vi "analysis_speech01.vi"(11 "文件路径（使用对话框）":path) -> (2 "数组":dbl[](array[numeric]), 3 "波形图表":waveform(dbl)[](graph))   [LabVIEW 2014]
uses:
  <vilib>/sound2/lvsound2.llb/Sound File Read Open.vi
  <vilib>/sound2/lvsound2.llb/Sound File Read (DBL).vi
panel:
  in  "布尔":bool
  out "错误输出":errorcluster
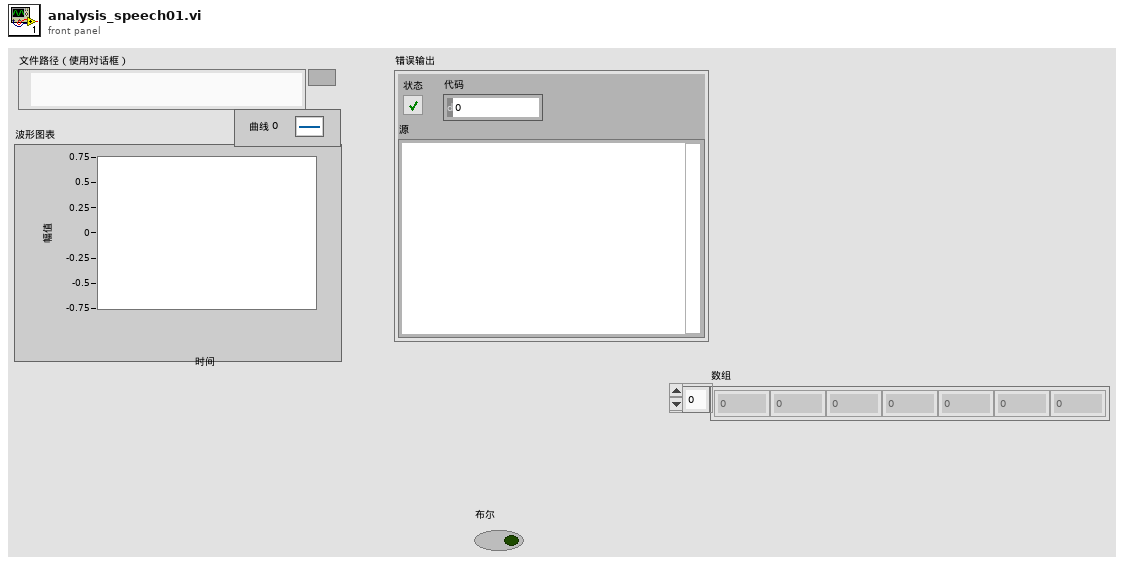
[diagram p1: front panel]
types:
  T1 = typedef "Sound File Refnum.ctl" = refnum<file>
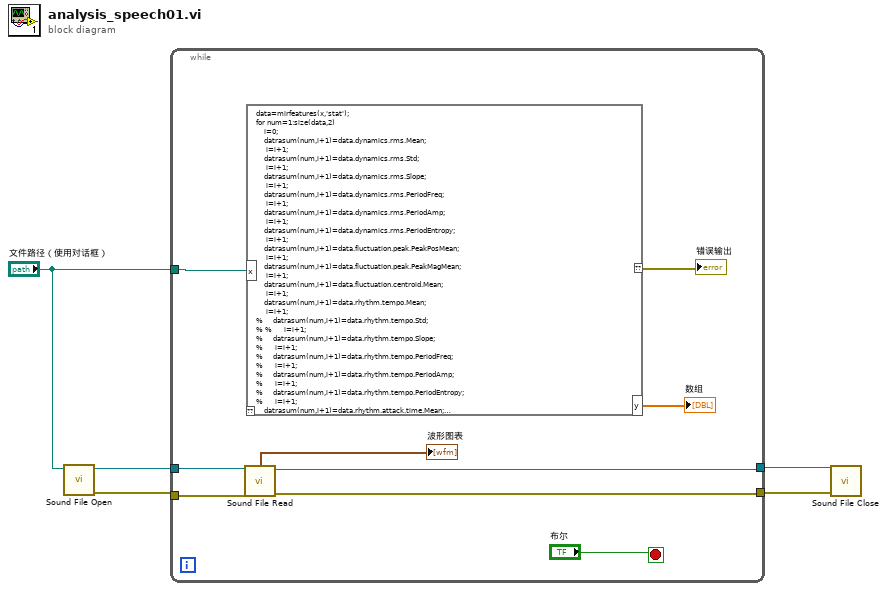
[diagram p0: block diagram]
diagram:
  n1 = call-poly <vilib>:"Sound File Open.vi"("path"="文件路径（使用对话框）") -> ("error out"=w2:errorcluster, "sound file refnum"=w4:T1)  [unwired: 9 in]
  n2 = while {
    tunnel: "文件路径（使用对话框）" -> [w10]
    tunnel: w4 -> [w11]
    tunnel: [w9] -> w3
    tunnel: w2 -> [w8]
    tunnel: [w7] -> w1
    stop <- "布尔" stop-if-true
    n3 = call-poly <vilib>:"Sound File Read.vi"("error in (no error)"=w8, "sound file refnum"=w11) -> ("error out"=w7:errorcluster, "data"=→"波形图表":waveform(dbl)[], "sound file refnum out"=w9:T1)  [unwired: 5 in, 2 out]
    n4 = script code="data=mirfeatures(x,'stat'); \nfor num=1:size(data,2)\n    i=0;\n    datrasum(num,i+1)=data.dynamics.rms.Mean;\n     i=i+1;\n    datrasum(num,i+1)=data.dynamics.rms.Std;\n     i=i+1;\n    datrasum(num,i+1)=data.dynamics.rms.Slope;\n     i=i+1;\n    datrasum(num,i+1)=data.dynamics.rms.PeriodFreq;\n     i=i+1;\n    datrasum(num,i+1)=data.dynamics.rms.PeriodAmp;\n     i=i+1;\n    datrasum(num,i+1)=data.dynamics.rms.PeriodEntropy;\n     i=i+1;\n    datrasum(num,i+1)=data.fluctuation.peak.PeakPosMean;\n     i=i+1;\n    datrasum(num,i+1)=data.fluctuation.peak.PeakMagMean;\n     i=i+1;\n    datrasum(num,i+1)=data.fluctuation.centroid.Mean;\n     i=i+1;\n    datrasum(num,i+1)=data.rhythm.tempo.Mean;\n     i=i+1;\n%     datrasum(num,i+1)=data.rhythm.tempo.Std;\n% %      i=i+1;\n%     datrasum(num,i+1)=data.rhythm.tempo.Slope;\n%      i=i+1;\n%     datrasum(num,i+1)=data.rhythm.tempo.PeriodFreq;\n%      i=i+1;\n%     datrasum(num,i+1)=data.rhythm.tempo.PeriodAmp;\n%      i=i+1;\n%     datrasum(num,i+1)=data.rhythm.tempo.PeriodEntropy;\n%      i=i+1;\n    datrasum(num,i+1)=data.rhythm.attack.time.Mean;\n     i=i+1;\n    datrasum(num,i+1)=data.rhythm.attack.time.Std;\n     i=i+1;\n    datrasum(num,i+1)=data.rhythm.attack.time.Slope;\n     i=i+1;\n    datrasum(num,i+1)=data.rhythm.attack.time.PeriodFreq;\n     i=i+1;\n    datrasum(num,i+1)=data.rhythm.attack.time.PeriodAmp;\n     i=i+1;\n    datrasum(num,i+1)=data.rhythm.attack.time.PeriodEntropy;\n     i=i+1;\n    datrasum(num,i+1)=data.rhythm.attack.slope.Mean;\n     i=i+1;\n    datrasum(num,i+1)=data.rhythm.attack.slope.Std;\n     i=i+1;\n    datrasum(num,i+1)=data.rhythm.attack.slope.Slope;\n     i=i+1;\n    datrasum(num,i+1)=data.rhythm.attack.slope.PeriodFreq;\n     i=i+1;\n    datrasum(num,i+1)=data.rhythm.attack.slope.PeriodAmp;\n     i=i+1;\n    datrasum(num,i+1)=data.rhythm.attack.slope.PeriodAmp;\n     i=i+1;\n    datrasum(num,i+1)=data.rhythm.attack.slope.PeriodEntropy;\n     i=i+1;\n    datrasum(num,i+1)=data.spectral.centroid.Mean;\n     i=i+1;\n    datrasum(num,i+1)=data.spectral.centroid.Std;\n     i=i+1;\n    datrasum(num,i+1)=data.spectral.centroid.Slope;\n     i=i+1;\n    datrasum(num,i+1)=data.spectral.centroid.PeriodFreq;\n     i=i+1;\n    datrasum(num,i+1)=data.spectral.centroid.PeriodAmp;\n     i=i+1;\n    datrasum(num,i+1)=data.spectral.centroid.PeriodEntropy;\n     i=i+1;\n    datrasum(num,i+1)=data.spectral.brightness.Mean;\n     i=i+1;\n    datrasum(num,i+1)=data.spectral.brightness.Std;\n     i=i+1;\n    datrasum(num,i+1)=data.spectral.brightness.Slope;\n     i=i+1;\n    datrasum(num,i+1)=data.spectral.brightness.PeriodFreq;\n     i=i+1;\n    datrasum(num,i+1)=data.spectral.brightness.PeriodAmp;\n     i=i+1;\n    datrasum(num,i+1)=data.spectral.brightness.PeriodEntropy;\n     i=i+1;\n    datrasum(num,i+1)=data.spectral.spread.Mean;\n     i=i+1;\n    datrasum(num,i+1)=data.spectral.spread.Std;\n     i=i+1;\n    datrasum(num,i+1)=data.spectral.spread.Slope;\n     i=i+1;\n    datrasum(num,i+1)=data.spectral.spread.PeriodFreq;\n     i=i+1;\n    datrasum(num,i+1)=data.spectral.spread.PeriodAmp;\n     i=i+1;\n    datrasum(num,i+1)=data.spectral.spread.PeriodEntropy;\n     i=i+1;\n    datrasum(num,i+1)=data.spectral.skewness.Mean;\n     i=i+1;\n    datrasum(num,i+1)=data.spectral.skewness.Std;\n     i=i+1;\n    datrasum(num,i+1)=data.spectral.skewness.Slope;\n     i=i+1;\n    datrasum(num,i+1)=data.spectral.skewness.PeriodFreq;\n     i=i+1;\n    datrasum(num,i+1)=data.spectral.skewness.PeriodAmp;\n     i=i+1;\n    datrasum(num,i+1)=data.spectral.skewness.PeriodEntropy;\n     i=i+1;\n    datrasum(num,i+1)=data.spectral.kurtosis.Mean;\n     i=i+1;\n    datrasum(num,i+1)=data.spectral.kurtosis.Std;\n     i=i+1;\n    datrasum(num,i+1)=data.spectral.kurtosis.Slope;\n     i=i+1;\n    datrasum(num,i+1)=data.spectral.kurtosis.PeriodFreq;\n     i=i+1;\n    datrasum(num,i+1)=data.spectral.kurtosis.PeriodAmp;\n     i=i+1;\n    datrasum(num,i+1)=data.spectral.kurtosis.PeriodEntropy;\n     i=i+1;\n    datrasum(num,i+1)=data.spectral.rolloff95.Mean;\n     i=i+1;\n    datrasum(num,i+1)=data.spectral.rolloff95.Std;\n     i=i+1;\n    datrasum(num,i+1)=data.spectral.rolloff95.Slope;\n     i=i+1;\n    datrasum(num,i+1)=data.spectral.rolloff95.PeriodFreq;\n     i=i+1;\n    datrasum(num,i+1)=data.spectral.rolloff95.PeriodAmp;\n     i=i+1;\n    datrasum(num,i+1)=data.spectral.rolloff95.PeriodEntropy;\n     i=i+1;\n    datrasum(num,i+1)=data.spectral.rolloff85.Mean;\n     i=i+1;\n    datrasum(num,i+1)=data.spectral.rolloff85.Std;\n     i=i+1;\n    datrasum(num,i+1)=data.spectral.rolloff85.Slope;\n     i=i+1;\n    datrasum(num,i+1)=data.spectral.rolloff85.PeriodFreq;\n     i=i+1;\n    datrasum(num,i+1)=data.spectral.rolloff85.PeriodAmp;\n     i=i+1;\n    datrasum(num,i+1)=data.spectral.rolloff85.PeriodEntropy;\n     i=i+1;\n    datrasum(num,i+1)=data.spectral.spectentropy.Mean;\n     i=i+1;\n    datrasum(num,i+1)=data.spectral.spectentropy.Std;\n     i=i+1;\n    datrasum(num,i+1)=data.spectral.spectentropy.Slope;\n     i=i+1;\n    datrasum(num,i+1)=data.spectral.spectentropy.PeriodFreq;\n     i=i+1;\n    datrasum(num,i+1)=data.spectral.spectentropy.PeriodAmp;\n     i=i+1;\n    datrasum(num,i+1)=data.spectral.spectentropy.PeriodEntropy;\n     i=i+1;\n    datrasum(num,i+1)=data.spectral.flatness.Mean;\n     i=i+1;\n    datrasum(num,i+1)=data.spectral.flatness.Std;\n     i=i+1;\n    datrasum(num,i+1)=data.spectral.flatness.Slope;\n     i=i+1;\n    datrasum(num,i+1)=data.spectral.flatness.PeriodFreq;\n     i=i+1;\n    datrasum(num,i+1)=data.spectral.flatness.PeriodAmp;\n     i=i+1;\n    datrasum(num,i+1)=data.spectral.flatness.PeriodEntropy;\n     i=i+1;\n    datrasum(num,i+1)=data.spectral.roughness.Mean;\n     i=i+1;\n    datrasum(num,i+1)=data.spectral.roughness.Std;\n     i=i+1;\n    datrasum(num,i+1)=data.spectral.roughness.Slope;\n     i=i+1;\n    datrasum(num,i+1)=data.spectral.roughness.PeriodFreq;\n     i=i+1;\n    datrasum(num,i+1)=data.spectral.roughness.PeriodAmp;\n     i=i+1;\n    datrasum(num,i+1)=data.spectral.roughness.PeriodEntropy;\n     i=i+1;\n    datrasum(num,i+1)=data.spectral.irregularity.Mean;\n     i=i+1;\n    datrasum(num,i+1)=data.spectral.irregularity.Std;\n     i=i+1;\n    datrasum(num,i+1)=data.spectral.irregularity.Slope;\n     i=i+1;\n    datrasum(num,i+1)=data.spectral.irregularity.PeriodFreq;\n     i=i+1;\n    datrasum(num,i+1)=data.spectral.irregularity.PeriodAmp;\n     i=i+1;\n    datrasum(num,i+1)=data.spectral.irregularity.PeriodEntropy; %mfcc为数组没有记录\n     i=i+1;\n    datrasum(num,i+1)=data.timbre.zerocross.Mean;\n     i=i+1;\n    datrasum(num,i+1)=data.timbre.zerocross.Std;\n     i=i+1;\n    datrasum(num,i+1)=data.timbre.zerocross.Slope;\n     i=i+1;\n    datrasum(num,i+1)=data.timbre.zerocross.PeriodFreq;\n     i=i+1;\n    datrasum(num,i+1)=data.timbre.zerocross.PeriodAmp;\n     i=i+1;\n    datrasum(num,i+1)=data.timbre.zerocross.PeriodEntropy;\n     i=i+1;\n    datrasum(num,i+1)=data.timbre.lowenergy.Mean;\n     i=i+1;\n    datrasum(num,i+1)=data.timbre.spectralflux.Mean;\n     i=i+1;\n    datrasum(num,i+1)=data.timbre.spectralflux.Std;\n     i=i+1;\n    datrasum(num,i+1)=data.timbre.spectralflux.Slope;\n     i=i+1;\n    datrasum(num,i+1)=data.timbre.spectralflux.PeriodFreq;\n     i=i+1;\n    datrasum(num,i+1)=data.timbre.spectralflux.PeriodAmp;\n     i=i+1;\n    datrasum(num,i+1)=data.timbre.spectralflux.PeriodEntropy;\n     i=i+1;\n    datrasum(num,i+1)=data.tonal.chromagram.peak.PeakPosMean;\n     i=i+1;\n    datrasum(num,i+1)=data.tonal.chromagram.peak.PeakPosStd;\n     i=i+1;\n    datrasum(num,i+1)=data.tonal.chromagram.peak.PeakPosSlope;\n     i=i+1;\n    datrasum(num,i+1)=data.tonal.chromagram.peak.PeakPosPeriodFreq ; %可能为nan\n     i=i+1;\n    datrasum(num,i+1)=data.tonal.chromagram.peak.PeakPosPeriodAmp ; %可能为nan\n     i=i+1;\n    datrasum(num,i+1)=data.tonal.chromagram.peak.PeakPosPeriodEntropy;\n     i=i+1;\n    datrasum(num,i+1)=data.tonal.chromagram.peak.PeakMagMean;\n     i=i+1;\n    datrasum(num,i+1)=data.tonal.chromagram.peak.PeakMagStd;\n     i=i+1;\n    datrasum(num,i+1)=data.tonal.chromagram.peak.PeakMagSlope;\n     i=i+1;\n    datrasum(num,i+1)=data.tonal.chromagram.peak.PeakMagPeriodFreq;\n     i=i+1;\n    datrasum(num,i+1)=data.tonal.chromagram.peak.PeakMagPeriodAmp;\n     i=i+1;\n    datrasum(num,i+1)=data.tonal.chromagram.peak.PeakMagPeriodEntropy;\n     i=i+1;\n    datrasum(num,i+1)=data.tonal.chromagram.centroid.Mean;\n     i=i+1;\n    datrasum(num,i+1)=data.tonal.chromagram.centroid.Std;\n     i=i+1;\n    datrasum(num,i+1)=data.tonal.chromagram.centroid.Slope;\n     i=i+1;\n    datrasum(num,i+1)=data.tonal.chromagram.centroid.PeriodFreq;\n     i=i+1;\n    datrasum(num,i+1)=data.tonal.chromagram.centroid.PeriodAmp;\n     i=i+1;\n    datrasum(num,i+1)=data.tonal.chromagram.centroid.PeriodEntropy;\n     i=i+1;\n    datrasum(num,i+1)=data.tonal.keyclarity.Mean;\n     i=i+1;\n    datrasum(num,i+1)=data.tonal.keyclarity.Std;\n     i=i+1;\n    datrasum(num,i+1)=data.tonal.keyclarity.Slope;\n     i=i+1;\n    datrasum(num,i+1)=data.tonal.keyclarity.PeriodFreq;\n     i=i+1;\n    datrasum(num,i+1)=data.tonal.keyclarity.PeriodAmp;\n     i=i+1;\n    datrasum(num,i+1)=data.tonal.keyclarity.PeriodEntropy;\n     i=i+1;\n    datrasum(num,i+1)=data.tonal.mode.Mean;\n     i=i+1;\n    datrasum(num,i+1)=data.tonal.mode.Std;\n     i=i+1;\n    datrasum(num,i+1)=data.tonal.mode.Slope;\n     i=i+1;\n    datrasum(num,i+1)=data.tonal.mode.PeriodFreq;\n     i=i+1;\n    datrasum(num,i+1)=data.tonal.mode.PeriodAmp;\n     i=i+1;\n    datrasum(num,i+1)=data.tonal.mode.PeriodEntropy;\n     i=i+1;\n    datrasum(num,i+1)=data.tonal.hcdf.Mean;\n     i=i+1;\n    datrasum(num,i+1)=data.tonal.hcdf.Std;\n     i=i+1;\n    datrasum(num,i+1)=data.tonal.hcdf.Slope;\n     i=i+1;\n    datrasum(num,i+1)=data.tonal.hcdf.PeriodFreq;\n     i=i+1;\n    datrasum(num,i+1)=data.tonal.hcdf.PeriodAmp;\n     i=i+1;\n    datrasum(num,i+1)=data.tonal.hcdf.PeriodEntropy;\n     i=i+1;\n\nend"("x"=w10) -> ("??"=→"错误输出":errorcluster, "y"=→"数组":cdb[])  [unwired: 1 in]
  }
  n5 = call <vilib>:"Sound File Close.vi"("error in (no error)"=w1, "sound file refnum"=w3) -> ()  [unwired: 9 in, 1 out]
